vi "niScope Fetch Cluster.vi"(7 "timeout":dbl=5.0 format="%.2f", 8 "error in":errorcluster, 9 "numSamples":i32=-1, 10 "channels":string="0", 11 "instrument handle":refnum<k15>) -> (0 "error out":errorcluster, 1 "waveform":T1 {"wfm" format="%.2f"; "xIncrement" format="%.2f"; "relativeInitialX" format="%.2f"}, 2 "wfm info":T2 {"reserved2" format="%.2f"; "reserved1" format="%.2f"; "offset" format="%^.3e"; "gain" format="%^.3e"; "xIncrement" format="%^.3e"; "relativeInitialX" format="%^.3e"; "absoluteInitialX" format="%^.3e"}, 3 "instrument handle out":refnum<k15>)   [LabVIEW 2013]
doc: "Retrieves the waveform the digitizer has acquired for the specified channel from a previously initiated acquisition. Returns scaled voltage waveforms in a cluster that includes timing information."
uses:
  niScope_32.dll
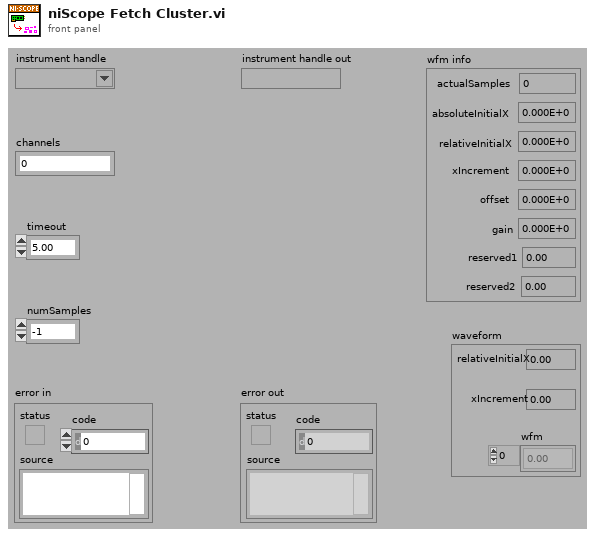
[diagram p1: front panel]
types:
  T1 = cluster{"relativeInitialX":dbl, "xIncrement":dbl, "wfm":dbl[]}
  T2 = cluster{"actualSamples":i32, "absoluteInitialX":dbl, "relativeInitialX":dbl, "xIncrement":dbl, "offset":dbl, "gain":dbl, "reserved1":dbl, "reserved2":dbl}
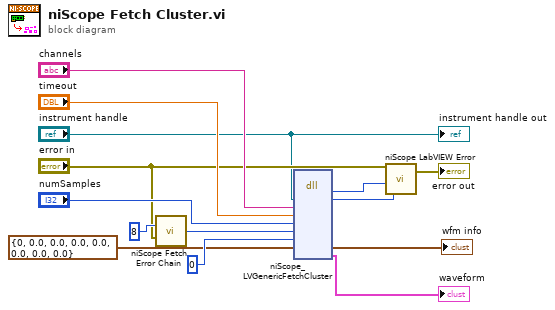
[diagram p0: block diagram]
diagram:
  n1 = call <instrlib>:"niScope Fetch Error Chain.vi"("dataType in"=8 ("dataType"), "error in"="error in") -> ("dataType"=w6:i32)  [unwired: 13 in]
  n2 = dll-call lib="niScope_*.*" fn="niScope_LVGenericFetchCluster"("instrument handle"="instrument handle", "channel"="channels", "timeout"="timeout", "numSamples"="numSamples", "dataType"=w6, "interleaved"=0 ("f"), "wfm_info"=T2 {"actualSamples"=0, "absoluteInitialX"=0.0, "relativeInitialX"=0.0, "xIncrement"=0.0, "offset"=0.0, "gain"=0.0, "reserved1"=0.0, "reserved2"=0.0} ("wfm info")) -> ("status"=w8:i32, "instrument handle"=w7:u32, "wfm_info"=→"wfm info":T2, "waveform"=→"waveform":T1)  [unwired: 9 in, 2 out]
  n3 = call <instrlib>:"niScope LabVIEW Error.vi"("instrument handle"=w7, "niScope error code (0)"=w8, "error in (no error)"="error in") -> ("error out"=→"error out":errorcluster)  [unwired: 2 in]
  "instrument handle out" <- "instrument handle"
